vi "segment.vi"(8 "error in (no error)":errorcluster, 9 "ImageCollection in":refnum<class "ImageCollection.lvclass">[](array[class]), 10 "image file path":path, 11 "SegmenterDL100224ThreeD in":refnum<class "SegmenterDL100224ThreeD.lvclass">) -> (0 "error out":errorcluster, 1 "ImageCollection out":refnum<class "ImageCollection.lvclass">[](array[class]), 2 "segmented image path":path, 3 "SegmenterDL100224ThreeD out":refnum<class "SegmenterDL100224ThreeD.lvclass">, 4 "centroids":T1[](array[typedef]))   [LabVIEW 2010, in "SegmenterDL100224ThreeD.lvclass"]
uses:
  SegmenterDL100224ThreeD.lvclass
  common/classes/ImageCollection/ImageCollection/ImageCollection.lvclass
  GenericSegmenter/GenericSegmenter/centroid_cluster.ctl
  <vilib>/Utility/file.llb/Read From Spreadsheet File (DBL).vi
  GenericSegmenter/GenericSegmenter/GenericSegmenter.lvclass
panel:
  out "console input":string
  out "console output":string
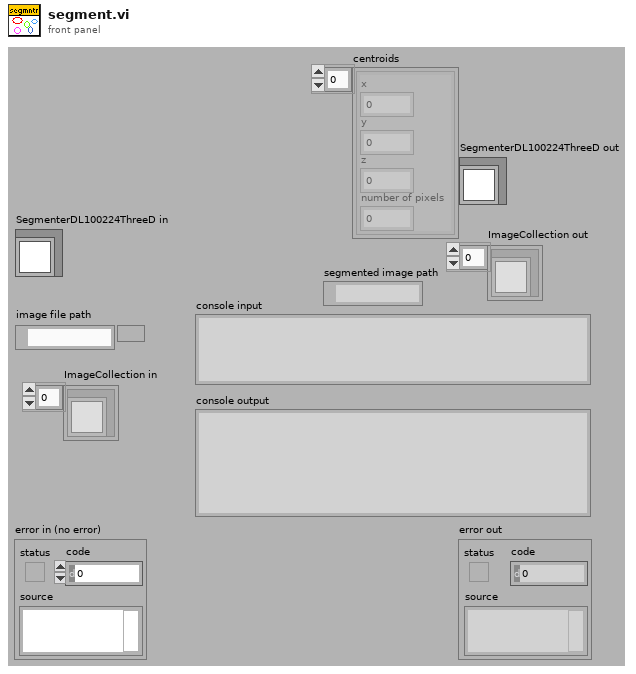
[diagram p1: front panel]
types:
  T1 = typedef "GenericSegmenter.lvclass/centroid_cluster.ctl" = cluster{"x":i32, "y":i32, "z":i32, "number of pixels":i32}
  T2 = cluster{"[0]":i32, "[1]":i32, "[2]":i32, "[3]":i32}
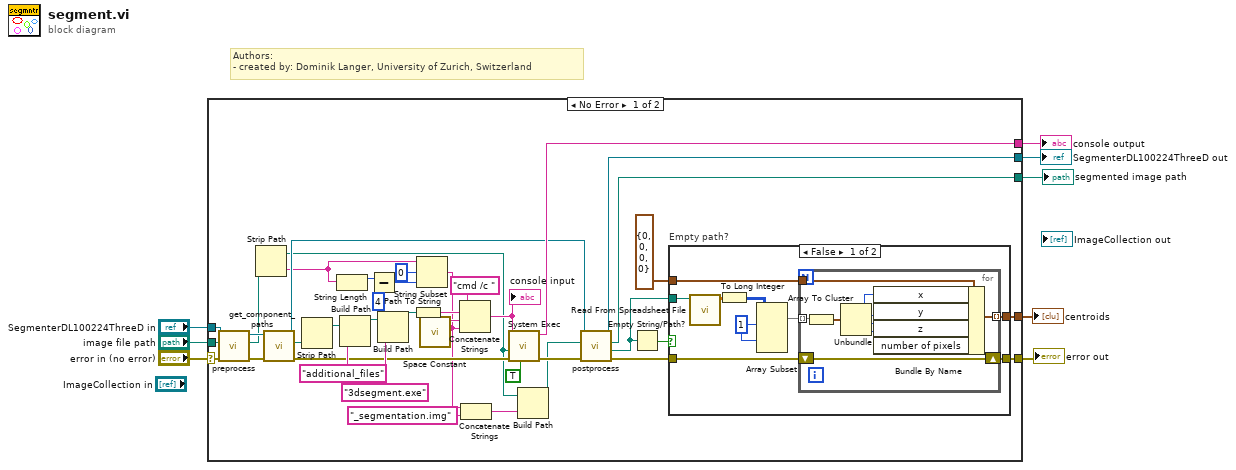
[diagram p0: block diagram]
diagram:
  # "Authors: \n- created by: Dominik Langer, University of Zurich, Switzerland"
  n1 = case shown="No Error" "error in (no error)" {
    selector: "error in (no error)" -> [w38 w68]
    tunnel: "SegmenterDL100224ThreeD in" -> [w36 w67]
    tunnel: [w11 w68] -> w6
    tunnel: [w23 w67] -> w5
    tunnel: "image file path" -> [w33 _]
    tunnel: [w31 _] -> w3
    tunnel: [w16 _] -> w2
    tunnel: [w10 _] -> w1
    frame No Error {
      n2 = call-dynamic "preprocess.vi"("error in (no error)"=w38, "image file path"=w33, "SegmenterDL100224ThreeD in"=w36) -> ("error out"=w37:errorcluster, "preprocessed file path"=w32:path, "SegmenterDL100224ThreeD out"=w34:refnum<class "SegmenterDL100224ThreeD.lvclass">)  [unwired: 6 in]
      n3 = Strip Path(path=w32) -> (stripped path=w17:path, name=w15:string)
      n4 = call-dynamic "get_component_paths.vi"("error in (no error)"=w37, "GenericComponent in"=w34) -> ("error out"=w40:errorcluster, "specific component directory"=w39:path, "GenericComponent out"=w24:refnum<class "SegmenterDL100224ThreeD.lvclass">)  [unwired: 4 in, 3 out]
      n5 = Strip Path(path=w39) -> (stripped path=w46:path)  [unwired: 1 out]
      n6 = String Length(string=w15) -> (length=w29:i32)
      n7 = Build Path(base path=w46, name or relative path="additional_files") -> (appended path=w44:path)
      n8 = Subtract(x=w29, y=4) -> (x-y=w27:i32)
      n9 = Build Path(base path=w44, name or relative path="3dsegment.exe") -> (appended path=w42:path)
      n10 = Path To String(path=w42) -> (string=w41:string)
      n11 = String Subset(string=w15, offset (0)=0, length (rest)=w27) -> (substring=w21:string)
      n12 = call <vilib>:"Space Constant.vi"() -> ("String"=w35:string)
      n13 = Concatenate Strings("cmd /c " ("string"), w41, w35, w21) -> (w25:string)
      "console input" <- w25
      n14 = Concatenate Strings(w21, "_segmentation.img" ("string")) -> (w18:string)
      n15 = call <vilib>:"System Exec.vi"("run minimized? (F)"=TRUE, "error in (no error)"=w40, "working directory"=w17, "command line"=w25) -> ("error out"=w22:errorcluster, "standard output"=w31:string)  [unwired: 4 in, 2 out]
      n16 = Build Path(base path=w17, name or relative path=w18) -> (appended path=w19:path)
      n17 = call-dynamic "postprocess.vi"("error in (no error)"=w22, "segmented image file path in"=w19, "SegmenterDL100224ThreeD in"=w24) -> ("error out"=w14:errorcluster, "centroids file path"=w13:path, "segmented image path out"=w16:path, "SegmenterDL100224ThreeD out"=w23:refnum<class "SegmenterDL100224ThreeD.lvclass">)  [unwired: 5 in]
      n18 = Empty String/Path?(string/path=w13) -> (empty?=w12:bool)
      n19 = case "Empty path?" shown="False" w12 {
        tunnel: w14 -> [w56 w66]
        tunnel: w13 -> [w53 _]
        tunnel: [w52 w66] -> w11
        tunnel: [w51 _] -> w10
        tunnel: T1 {"x"=0, "y"=0, "z"=0, "number of pixels"=0} ("centroid") -> [w48 _]
        frame False {
          w55 = 1 ("index")
          n20 = call-poly <vilib>:"Read From Spreadsheet File.vi"("file path (dialog if empty)"=w53) -> ("all rows"=w50:dbl[][])  [unwired: 6 in, 4 out]
          n21 = To Long Integer(number=w50) -> (32bit integer=w49:i32[][])
          n22 = Array Subset(array=w49, index (row)=w55, index (col)=w55) -> (w54:i32[][])  [unwired: 2 in]
          n23 = for {
            tunnel: w54 -> [w62] mode=indexing
            shift-right: [w65] -> w52
            shift-left: w56 -> [w65]
            tunnel: [w63] -> w51 mode=indexing
            tunnel: w48 -> [w64]
            n24 = Array To Cluster(array=w62) -> (cluster=w61:T2)
            n25 = Unbundle(w61) -> ("[0]"=w60:i32, "[1]"=w59:i32, "[2]"=w58:i32, "[3]"=w57:i32)
            n26 = Bundle By Name(cluster=w64, "x"=w60, "y"=w59, "z"=w58, "number of pixels"=w57) -> (w63:T1)
          }
        }
        frame True {
        }
      }
    }
    frame Error {
    }
  }
  "error out" <- w6
  "SegmenterDL100224ThreeD out" <- w5
  "console output" <- w3
  "segmented image path" <- w2
  "centroids" <- w1
